vi "trio_test.vi"() -> ()   [LabVIEW 2017]
uses:
  <instrlib>/Trio Motion/Trio Motion Library.lvlib
panel:
  out "Reverse Limit":bool
  out "Forward Limit":bool
  out "MoveRel":bool
  in  "Distance":dbl format="%#_13g"
  in  "Move rel":bool
  in  "Axis":i16
  in  "Variable":string
  out "Value":dbl=-1.0 format="%#_13g"
  out "Read Param":bool
  out "error out":errorcluster
  in  "stop":bool
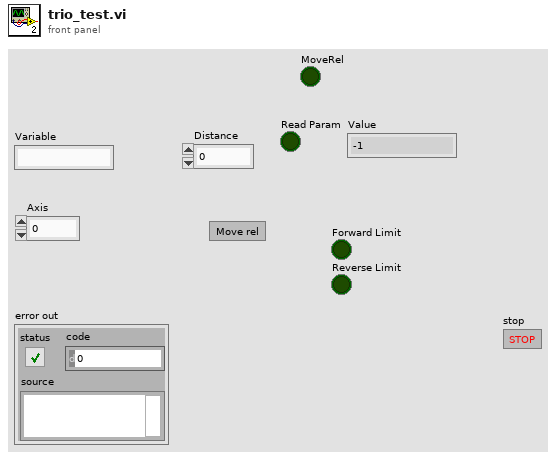
[diagram p1: front panel]
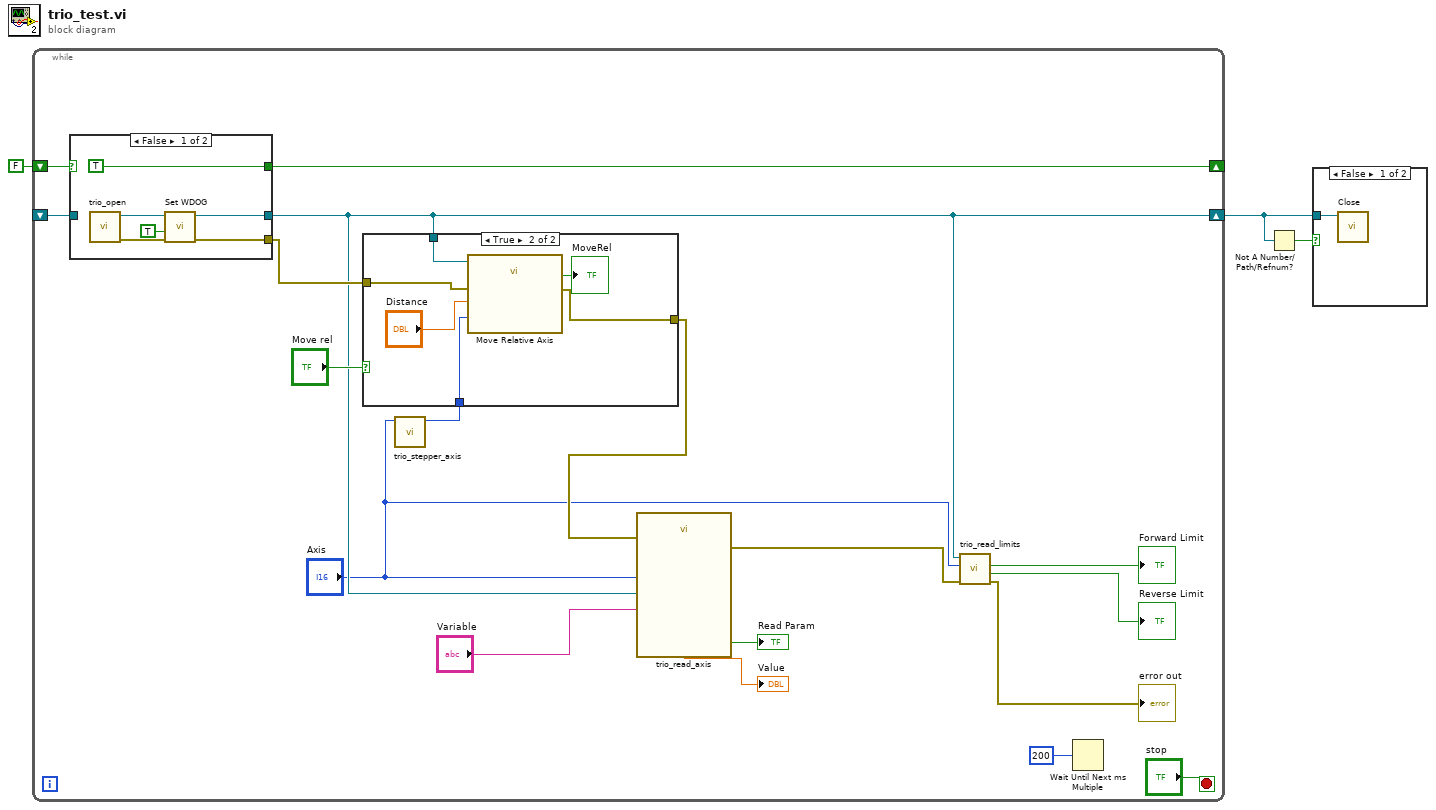
[diagram p0: block diagram]
diagram:
  n1 = while {
    shift-right: [w19] -> _
    shift-left: FALSE -> [w20]
    shift-right: [w9] -> w3
    shift-left: _ -> [w18]
    stop <- "stop" stop-if-true
    n2 = case shown="False" w20 {
      selector: w20 -> [_ w35]
      tunnel: [TRUE w35] -> w19
      tunnel: [w29 w36] -> w9
      tunnel: w18 -> [_ w36]
      tunnel: [w30 _] -> w12
      frame False {
        n3 = call "trio_open.vi"() -> ("error out"=w32:errorcluster, "reference out"=w31:refnum<k7>)  [unwired: 10 in]
        n4 = call <instrlib>:"Set WDOG.vi"("error in (no error)"=w32, "WDOG (ON)"=TRUE, "reference in"=w31) -> ("error out"=w30:errorcluster, "reference out"=w29:refnum<k7>)  [unwired: 6 in, 1 out]
      }
      frame True {
      }
    }
    n5 = call "trio_stepper_axis.vi"("Encoder axis"="Axis") -> ("Stepper axis"=w7:i32)  [unwired: 10 in]
    n6 = case shown="True" "Move rel" {
      tunnel: w9 -> [_ w27]
      tunnel: w12 -> [w22 w25]
      tunnel: [w22 w24] -> w11
      tunnel: w7 -> [_ w23]
      frame False {
      }
      frame True {
        n7 = call <instrlib>:"Move Relative Axis.vi"("error in (no error)"=w25, "Distance"="Distance", "Axis (0)"=w23, "reference in"=w27) -> ("error out"=w24:errorcluster, "MoveRel"=→"MoveRel":bool)  [unwired: 5 in, 1 out]
      }
    }
    n8 = call "trio_read_axis.vi"("Axis"="Axis", "error in (no error)"=w11, "Variable"="Variable", "reference in"=w9) -> ("error out"=w8:errorcluster, "Value"=→"Value":dbl, "GetAxisVariable"=→"Read Param":bool)  [unwired: 5 in]
    n9 = call "trio_read_limits.vi"("error in (no error)"=w8, "Axis"="Axis", "Trio ref in"=w9) -> ("error out"=→"error out":errorcluster, "Reverse Limit"=→"Reverse Limit":bool, "Forward Limit"=→"Forward Limit":bool)  [unwired: 5 in, 1 out]
    n10 = Wait Until Next ms Multiple(millisecond multiple=u32 200) -> ()  [unwired: 1 out]
  }
  n11 = Not A Number/Path/Refnum?(number/path/refnum=w3) -> (NaN/Path/Refnum?=w2:bool)
  n12 = case shown="False" w2 {
    tunnel: w3 -> [w37 _]
    frame False {
      n13 = call <instrlib>:"Close.vi"("reference in"=w37) -> ()  [unwired: 10 in, 1 out]
    }
    frame True {
    }
  }
